vi "Fishing OCR.vi"() -> ()   [LabVIEW 2019]
panel:
  out "Input":picture
  out "String Output":string
  out "Filtered String Output":string
  in  "error in":errorcluster
  out "OCR Post-Process Output":T1(plugin-control)
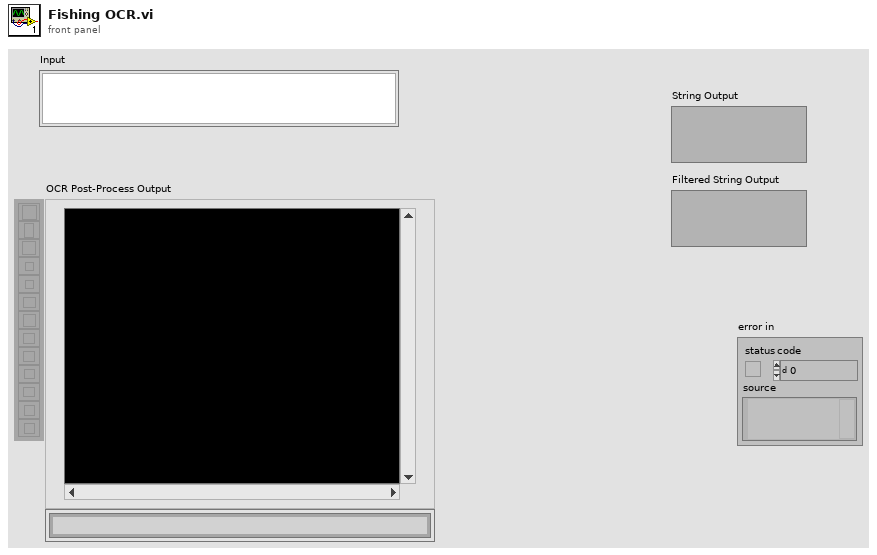
[diagram p1: front panel]
types:
  T1 = typedef "IMAQ Image.ctl" = refnum<image>
  T2 = typedef "Image Type" = u32
  T3 = typedef "imagedata.ctl" = cluster{"image type":i32, "image depth":i32, "image":u8[], "mask":u8[], "colors":u32[], "Rectangle":cluster{"left":i16, "top":i16, "right":i16, "bottom":i16}}
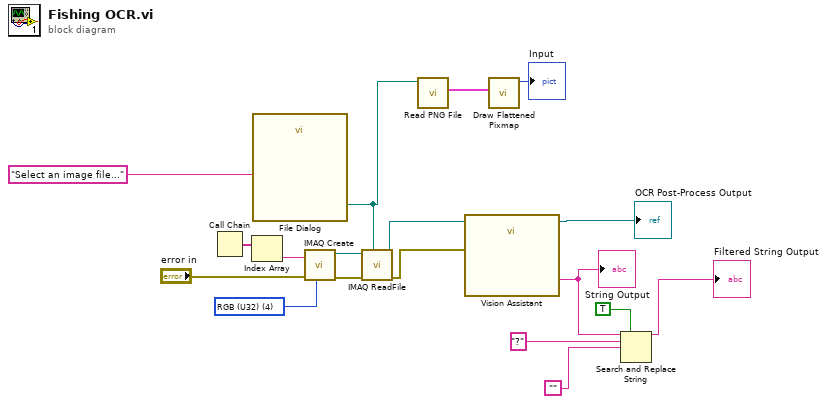
[diagram p0: block diagram]
diagram:
  w12 = T2 4 items=["Grayscale (U8)", "Grayscale (I16)", "Grayscale (SGL)", "Complex (CSG)", "RGB (U32)", "HSL (U32)", "RGB (U64)", "Grayscale (U16)"] ("Image Type")
  n1 = Call Chain() -> (call chain=w15:string[])
  n2 = Index Array(array=w15) -> (element=w14:string)  [unwired: 1 in]
  n3 = call "File Dialog"("prompt"="Select an image file...") -> ("selected path"=w2:path)  [unwired: 6 in, 8 out]
  n4 = call "IMAQ Create"("Image Name"=w14, "Image Type"=w12, "error in (no error)"="error in") -> ("New Image"=w18:T1, "error out"=w17:errorcluster)  [unwired: 1 in, 1 out]
  n5 = call "IMAQ ReadFile"("File Path"=w2, "error in (no error)"=w17, "Image"=w18) -> ("error out"=w10:errorcluster, "Image Out"=w4:T1)  [unwired: 2 in, 5 out]
  n6 = call <vilib>:"Read PNG File.vi"("path to PNG file"=w2) -> ("image data"=w1:T3)  [unwired: 8 in, 2 out]
  n7 = call "Vision Assistant"("Image In"=w4, "error in"=w10) -> ("Image Out"=→"OCR Post-Process Output":T1, "String (OCR/OCV 2)"=w6:string)  [unwired: 23 in, 1 out]
  "String Output" <- w6
  n8 = call <vilib>:"Draw Flattened Pixmap.vi"("image data"=w1) -> ("new picture"=→"Input":picture)  [unwired: 8 in]
  n9 = Search and Replace String(replace all?=TRUE ("replace all? (F)"), input string=w6, search string="?", replace string="") -> (result string=→"Filtered String Output":string)  [unwired: 4 in, 3 out]
